vi "Log Message.vi"(4 "Actor Name":string, 5 "Level":T1, 6 "Actor Type":string, 8 "error in (no error)":errorcluster, 11 "Message":string) -> (0 "error out":errorcluster)   [LabVIEW 2016, in "Stream Log.lvlib" / "Global Application Log.lvclass"]
doc: "--\nCopyright © 2017 Composed SystemsI All rights reserved.\n\nAuthor: Jon McBee <jon.mcbee@composed.io>\n\nThis library is provided \"AS IS\" ,WITHOUT WARRANTIES OR\nCONDITIONS OF ANY KIND, either express or implied.\n\nComposed Systems -- composed.io\n\nStream 0.0.1.1\nJon McBee - Composed Systems\nCopyright (c) 2017, Composed Systems"
uses:
  <userlib>/Composed Systems/Stream/Log/Global Application Log/Global Application Log.lvclass
  <userlib>/Composed Systems/Stream/Log/Application Log/Log Level.ctl
  <userlib>/Composed Systems/Stream/Log/Global Application Log/Global Application Log.lvclass/Global Application Log.ctl
  <userlib>/Composed Systems/Stream/Log/Application Log/Application Log.lvclass
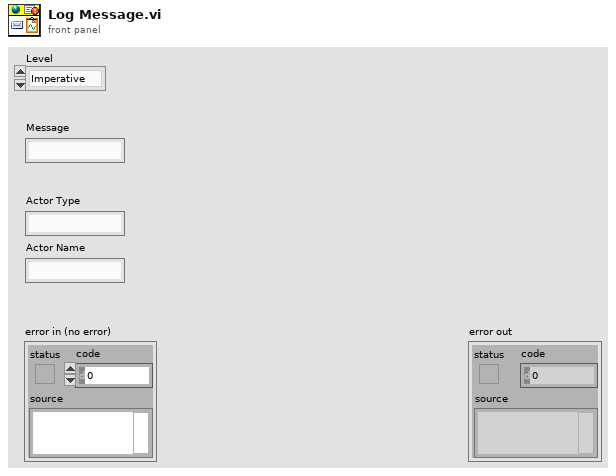
[diagram p1: front panel]
types:
  T1 = typedef "Stream Log.lvlib/Application Log.lvclass/Log Level.ctl" = enum16{"Imperative", "Major", "Minor", "Debug", "Off"}
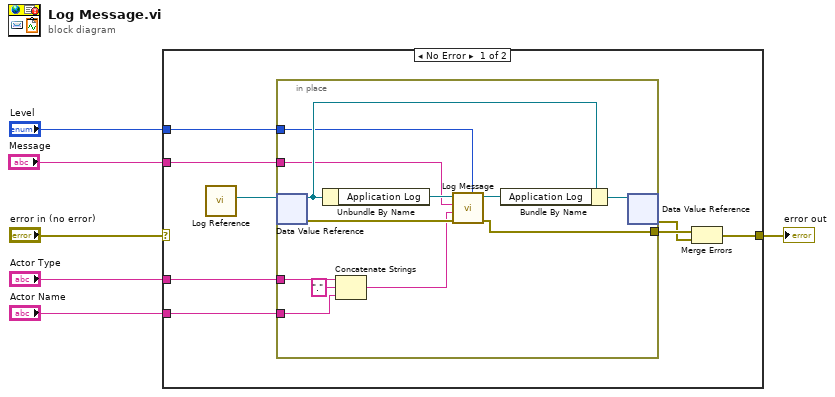
[diagram p0: block diagram]
diagram:
  n1 = case shown="No Error" "error in (no error)" {
    selector: "error in (no error)" -> [_ w27]
    tunnel: [w7 w27] -> w5
    tunnel: "Level" -> [w11 _]
    tunnel: "Message" -> [w10 _]
    tunnel: "Actor Type" -> [w9 _]
    tunnel: "Actor Name" -> [w8 _]
    frame No Error {
      n2 = call <userlib>:"Log Reference.vi"() -> ("Global Log Reference out"=w14:refnum<data-value>)  [unwired: 11 in]
      n3 = in-place {
        in-place-border: [w21] -> w13
        in-place-border: w11 -> [w20]
        in-place-border: w10 -> [w19]
        in-place-border: w9 -> [w18]
        in-place-border: w8 -> [w17]
        n4 = in-place-dvr #1(w14) -> (w26:refnum<class "Global Application Log.lvclass">, w22:errorcluster)
        n5 = Unbundle By Name(w26) -> ("Application Log"=w24:refnum<class "Application Log.lvclass">)
        n6 = Concatenate Strings(w18, "." ("string"), w17) -> (w15:string)
        n7 = call <userlib>:"Log Message.vi"("Level"=w20, "error in (no error)"=w22, "Actor Type.Name"=w15, "Message"=w19, "Application Log in"=w24) -> ("error out"=w21:errorcluster, "Application Log out"=w23:refnum<class "Application Log.lvclass">)  [unwired: 5 in]
        n8 = Bundle By Name(cluster=w26, "Application Log"=w23) -> (w25:refnum<class "Global Application Log.lvclass">)
        n9 = in-place-dvr #1(w25) -> (w12:errorcluster)  [unwired: 1 out]
      }
      n10 = Merge Errors(w13, w12) -> (w7:errorcluster)
    }
    frame Error {
    }
  }
  "error out" <- w5
